vi "Simple_template.vi"(9 "Angle1":dbl(knob)=-45.83837436417874 scale=-90.0..90.0, 11 "L 1":dbl(slide)=80.0 scale=0.0..200.0) -> (3 "2D Picture":picture)   [LabVIEW 2024]
panel:
  # "A 2"
  # "L1"
  # "L2"
  # "A 1"
  # "mm"
  # "mm"
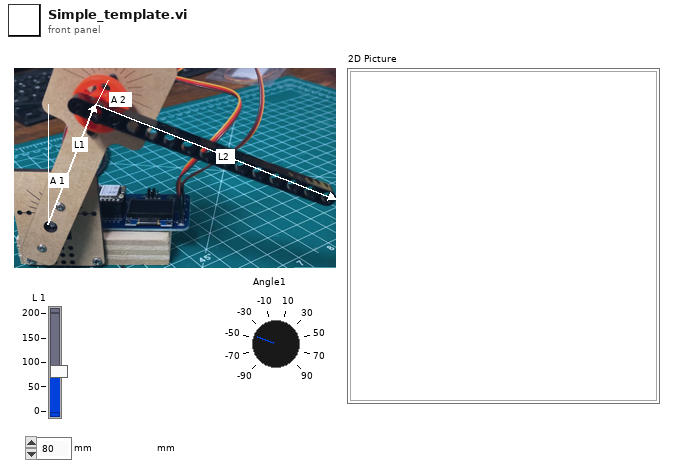
[diagram p1: front panel]
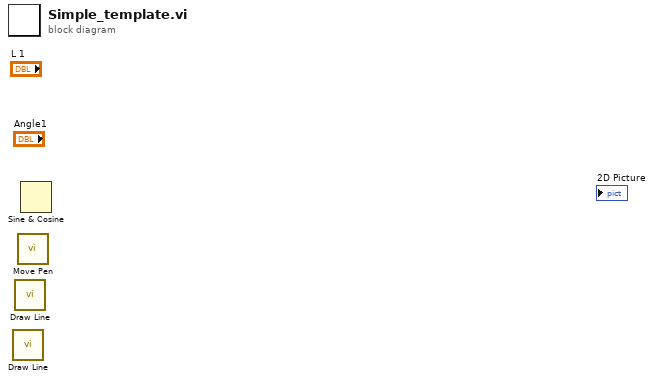
[diagram p0: block diagram]
diagram:
  n1 = call <vilib>:"Draw Line.vi"() -> ()  [unwired: 9 in, 1 out]
  n2 = call <vilib>:"Draw Line.vi"() -> ()  [unwired: 9 in, 1 out]
  n3 = call <vilib>:"Move Pen.vi"() -> ()  [unwired: 5 in, 1 out]
  n4 = Sine & Cosine() -> ()  [unwired: 1 in, 2 out]
